vi "Open MSG for SMU.vi"(9 "timeout in ms (-1)":i32=-1, 10 "Initialized":bool, 11 "Queue in":T1) -> (0 "error out":errorcluster, 1 "Unread":i32, 2 "Data":variant, 3 "Command":T2)   [LabVIEW 2018, in "Source meter.lvlib"]
uses:
  Source meter.lvlib
  ctls/SMU Commands.ctl
  Messenger service/Data types/Mailbox address.ctl
  ctls/MSG to SMU.ctl
  Messenger service/MessengerLib.lvlib
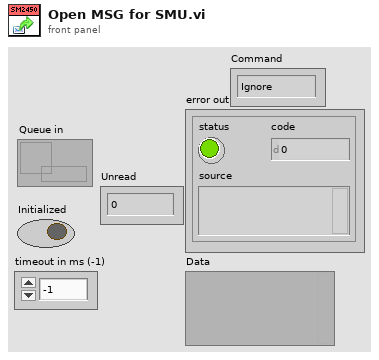
[diagram p1: front panel]
types:
  T1 = typedef "MessengerLib.lvlib/Mailbox address.ctl" = refnum<queue>
  T2 = typedef "Source meter.lvlib/SMU Commands.ctl" = enum16{"Ignore", "Connect", "Update", "Set measurement", "Start measurement", "Get actual results", "Stop measurement", "Disconnect", "End"}
  T3 = typedef "Source meter.lvlib/MSG to SMU.ctl" = cluster{"Command":T2, "Data":variant}
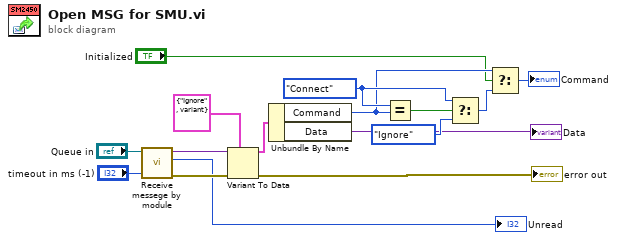
[diagram p0: block diagram]
diagram:
  w12 = SMU_Commands."Connect" ("Command")
  n1 = call "Receive messege by module.vi"("timeout in ms (-1)"="timeout in ms (-1)", "Module mailbox"="Queue in") -> ("error out"=w6:errorcluster, "Unread"=→"Unread":i32, "Data"=w1:variant)  [unwired: 5 in, 2 out]
  n2 = Variant To Data(error in=w6, type=T3 {"Command"=enum."Ignore", "Data"=variant} ("MSG to Source meter"), Variant=w1) -> (data=w10:T3, error out=→"error out":errorcluster)
  n3 = Unbundle By Name(w10) -> ("Command"=w11:T2, "Data"=→"Data":variant)
  n4 = Equal?(x=w12, y=w11) -> (x = y?=w13:bool)
  n5 = Select(t=w12, s=w13, f=SMU_Commands."Ignore" ("Command")) -> (s? t:f=w14:T2)
  n6 = Select(t=w11, s="Initialized", f=w14) -> (s? t:f=→"Command":T2)
